vi "telemetry_subscriber.vi"() -> ()   [LabVIEW 2016]
uses:
  ts_sallv_exa/DataTypes/Timestamp.ctl
  ts_sallv_exa/SALLV_EXA.lvlib
panel:
  out "Looptime":dbl(graph)
  out "Time":T1
  out "Count":i32
  out "Stop 2":bool=TRUE
  out "Stop":bool=TRUE
  in  "stop":bool
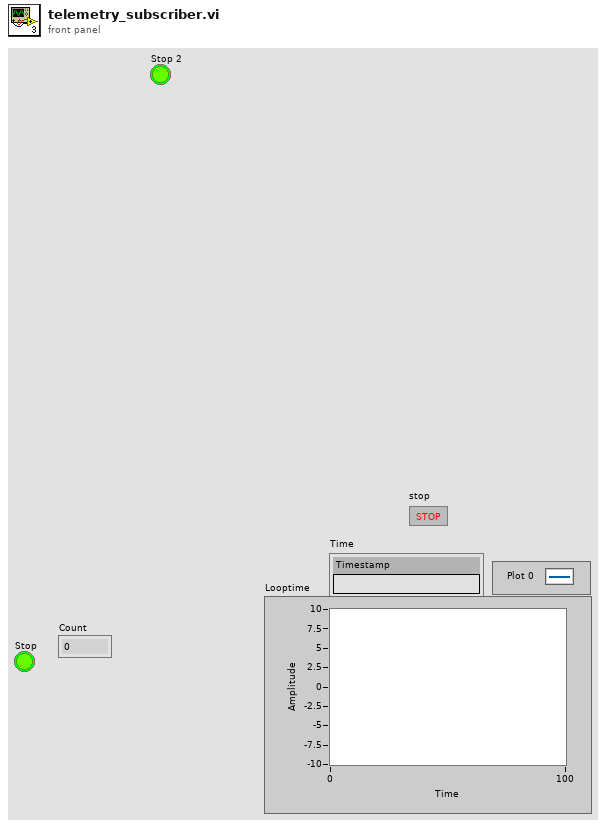
[diagram p1: front panel]
types:
  T1 = typedef "SALLV_EXA.lvlib/Timestamp.ctl" = cluster{"Timestamp":string}
  T2 = typedef "SALLV_EXA.lvlib/LoopTime_ms.ctl" = cluster{"LoopTime_ms":dbl}
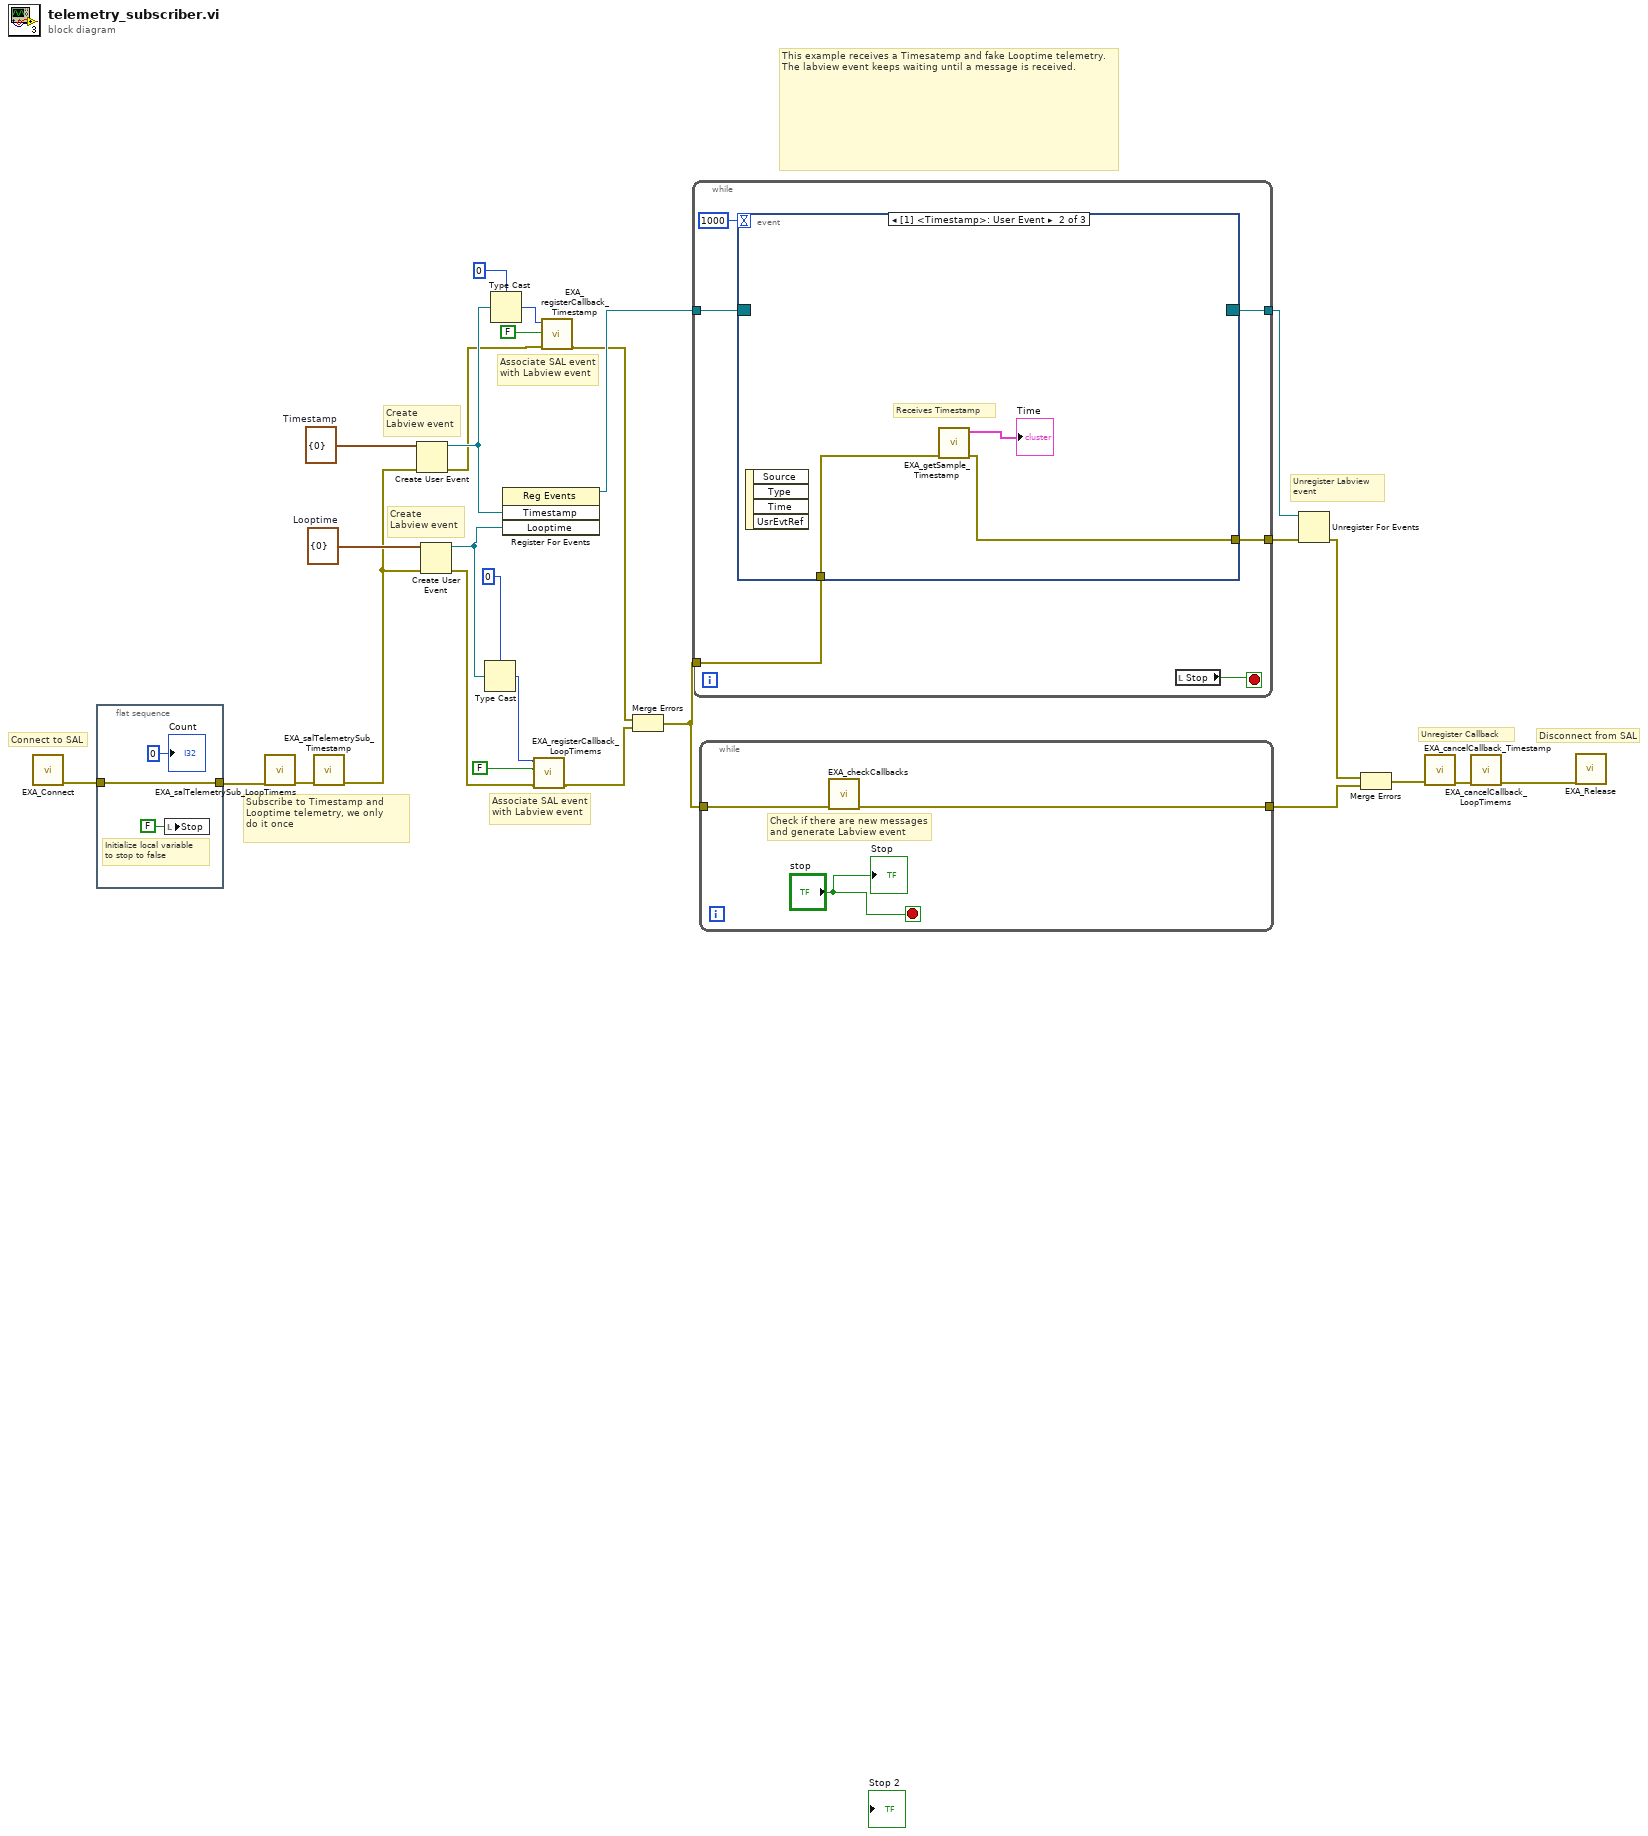
[diagram p0: block diagram]
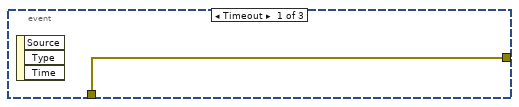
[diagram p2: hidden frame]
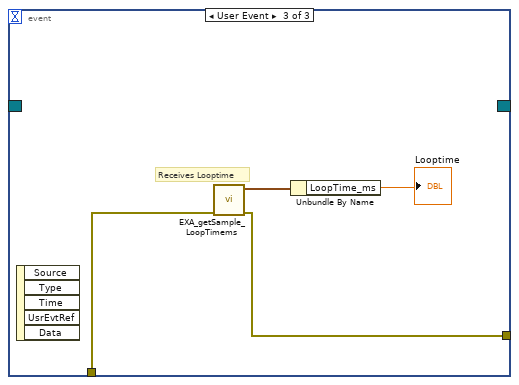
[diagram p3: hidden frame]
diagram:
  w19 = cluster{"Data":i32} {"Data"=0}  # Timestamp
  w26 = cluster{"Data":i32} {"Data"=0}  # Looptime
  # "Create Labview event"
  # "Associate SAL event\nwith Labview event"
  # "This example receives a Timesatemp and fake Looptime telemetry. The labview event keeps waiting until a message is received."
  # "Unregister Labview\nevent"
  # "Create Labview event"
  # "Associate SAL event\nwith Labview event"
  # "Unregister Callback"
  # "Subscribe to Timestamp and Looptime telemetry, we only\ndo it once"
  # "Disconnect from SAL"
  # "Connect to SAL"
  n1 = call "EXA_Connect.vi"() -> ("error out"=w27:errorcluster)  [unwired: 10 in, 1 out]
  n2 = flat-sequence {
    tunnel: w27 -> [w29]
    tunnel: [w29] -> w12
    frame #0 {
      # "Initialize local variable \nto stop to false"
      n3 = local write "Stop"(FALSE ("Stop")) -> ()
      "Count" <- 0 ("Count")
    }
  }
  n4 = call "EXA_salTelemetrySub_LoopTimems.vi"("error in (no error)"=w12) -> ("error out"=w13:errorcluster)  [unwired: 9 in, 1 out]
  n5 = call "EXA_salTelemetrySub_Timestamp.vi"("error in (no error)"=w13) -> ("error out"=w14:errorcluster)  [unwired: 9 in, 1 out]
  n6 = Create User Event(user event datatype=w19, error in=w14) -> (user event=w16:refnum<user-event>, error out=w11:errorcluster)
  n7 = Create User Event(user event datatype=w26, error in=w14) -> (user event=w18:refnum<user-event>, error out=w5:errorcluster)
  n8 = Type Cast(type=0 ("handle"), x=w18) -> (*(type *) &x=w7:i32)
  n9 = Type Cast(type=0 ("handle"), x=w16) -> (*(type *) &x=w8:i32)
  n10 = register-events(w16, w18) -> (reference out=w24:refnum<event-registration>)  [unwired: 2 in, 1 out]
  n11 = call "EXA_registerCallback_LoopTimems.vi"("error in (no error)"=w5, "skipOld"=FALSE, "handle"=w7) -> ("error out"=w4:errorcluster)  [unwired: 7 in, 1 out]
  n12 = call "EXA_registerCallback_Timestamp.vi"("error in (no error)"=w11, "skipOld"=FALSE, "handle"=w8) -> ("error out"=w10:errorcluster)  [unwired: 7 in, 1 out]
  n13 = Merge Errors(w10, w4) -> (w15:errorcluster)
  n14 = while {
    tunnel: w24 -> [w34]
    tunnel: w15 -> [w33]
    tunnel: [w32] -> w22
    tunnel: [w31] -> w21
    stop <- w36 stop-if-true
    n15 = event shown="[1] <Timestamp>: User Event" {
      selector: w34 -> [_ _ _]
      dyn-events: [_ _ _] -> w31
      timeout: 1000 -> [_ _ _]
      tunnel: w33 -> [w37 w40 w43]
      tunnel: [w37 w39 w44] -> w32
      event Timeout {
        n16 = event-data() -> ()  [unwired: 1 in, 3 out]
      }
      event User Event {
        # "Receives Timestamp"
        n17 = event-data() -> ()  [unwired: 1 in, 4 out]
        n18 = call "EXA_getSample_Timestamp.vi"("error in (no error)"=w40) -> ("error out"=w39:errorcluster, "Timestamp_Ctl out"=→"Time":T1)  [unwired: 8 in, 1 out]
      }
      event User Event {
        # "Receives Looptime"
        n19 = event-data() -> ()  [unwired: 1 in, 5 out]
        n20 = call "EXA_getSample_LoopTimems.vi"("error in (no error)"=w43) -> ("error out"=w44:errorcluster, "LoopTime_ms_Ctl out"=w42:T2)  [unwired: 8 in, 1 out]
        n21 = Unbundle By Name(w42) -> ("LoopTime_ms"=→"Looptime":dbl)
      }
    }
    n22 = local read "Stop"() -> (w36:bool)
  }
  n23 = while {
    tunnel: w15 -> [w46]
    tunnel: [w45] -> w23
    stop <- "stop" stop-if-true
    # "Check if there are new messages \nand generate Labview event"
    n24 = call "EXA_checkCallbacks.vi"("error in (no error)"=w46) -> ("error out"=w45:errorcluster)  [unwired: 10 in]
    "Stop" <- "stop"
  }
  n25 = Unregister For Events(event registration refnum=w21, error in=w22) -> (error out=w20:errorcluster)
  n26 = Merge Errors(w20, w23) -> (w3:errorcluster)
  n27 = call "EXA_cancelCallback_Timestamp.vi"("error in (no error)"=w3) -> ("error out"=w2:errorcluster)  [unwired: 9 in, 1 out]
  n28 = call "EXA_cancelCallback_LoopTimems.vi"("error in (no error)"=w2) -> ("error out"=w1:errorcluster)  [unwired: 9 in, 1 out]
  n29 = call "EXA_Release.vi"("error in (no error)"=w1) -> ()  [unwired: 9 in, 2 out]
